vi "Parse Next XML Tag.vi"(8 "error in (no error)":errorcluster, 11 "XML in":string) -> (0 "error out":errorcluster, 1 "Tag":string, 2 "Before Tag":string, 3 "XML out":string)   [LabVIEW 2017, in "Feed.lvclass"]
uses:
  <vilib>/NI_RSS/Feed/Feed.lvclass
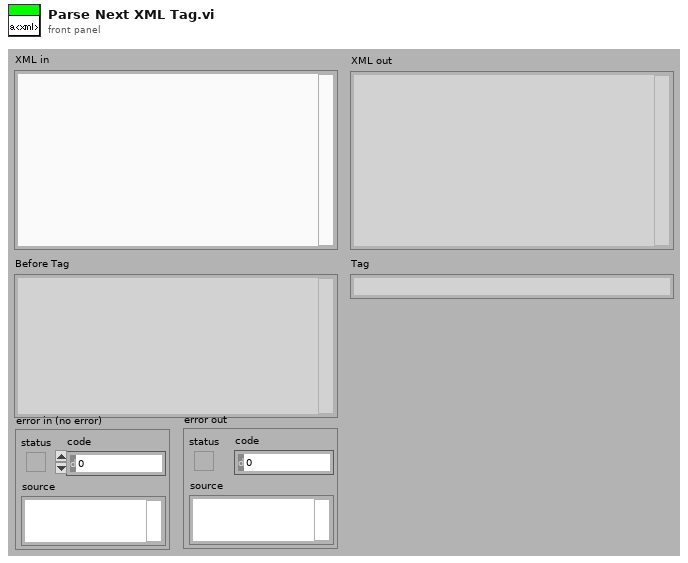
[diagram p1: front panel]
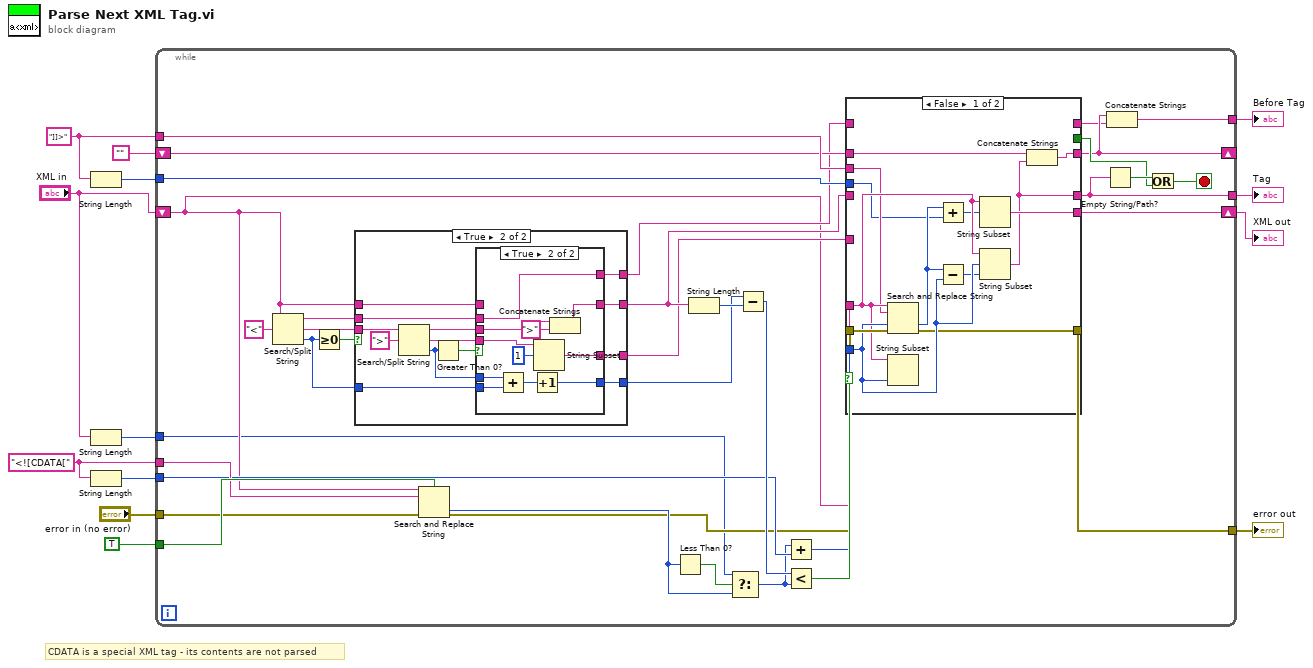
[diagram p0: block diagram]
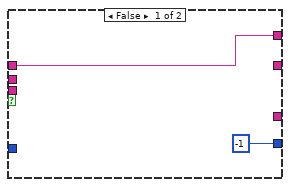
[diagram p2: hidden frame]
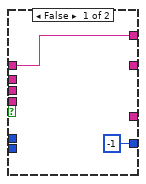
[diagram p3: hidden frame]
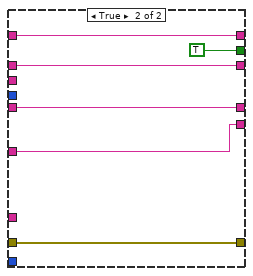
[diagram p4: hidden frame]
diagram:
  w4 = "]]>" ("regular expression")
  w6 = "<![CDATA[" ("regular expression")
  # "CDATA is a special XML tag - its contents are not parsed"
  n1 = String Length(string=w4) -> (length=w3:i32)
  n2 = String Length(string="XML in") -> (length=w1:i32)
  n3 = String Length(string=w6) -> (length=w5:i32)
  n4 = while {
    tunnel: TRUE ("ignore case? (F)") -> [w48]
    tunnel: w6 -> [w36]
    tunnel: "error in (no error)" -> [w46]
    tunnel: [w32] -> w11
    tunnel: [w41] -> w10
    tunnel: [w42] -> w8
    shift-right: [w43] -> w9
    shift-left: "XML in" -> [w15]
    shift-right: [w34] -> _
    shift-left: "" -> [w35]
    tunnel: w4 -> [w37]
    tunnel: w5 -> [w31]
    tunnel: w3 -> [w29]
    tunnel: w1 -> [w14]
    stop <- w38 stop-if-true
    n5 = Search/Split String(string=w15, search string/char (-)="<") -> (substring before match=w21:string, match + rest of string=w22:string, offset of match=w20:i32)  [unwired: 1 in]
    n6 = Greater Or Equal To 0?(x=w20) -> (x >= 0?=w23:bool)
    n7 = case shown="True" w23 {
      tunnel: w22 -> [_ w63]
      tunnel: w21 -> [_ w57]
      tunnel: w15 -> [w50 w58]
      tunnel: [_ w54] -> w18
      tunnel: [w50 w56] -> w19
      tunnel: [_ w55] -> w17
      tunnel: w20 -> [_ w52]
      tunnel: [-1 w51] -> w16
      frame False {
      }
      frame True {
        n8 = Search/Split String(string=w63, search string/char (-)=">") -> (substring before match=w59:string, match + rest of string=w60:string, offset of match=w53:i32)  [unwired: 1 in]
        n9 = Greater Than 0?(x=w53) -> (x > 0?=w61:bool)
        n10 = case shown="True" w61 {
          tunnel: w60 -> [_ w75]
          tunnel: w59 -> [_ w72]
          tunnel: w58 -> [w65 _]
          tunnel: w57 -> [_ w76]
          tunnel: [w65 w76] -> w56
          tunnel: [_ w73] -> w55
          tunnel: [_ w70] -> w54
          tunnel: w53 -> [_ w68]
          tunnel: w52 -> [_ w67]
          tunnel: [-1 w66] -> w51
          frame False {
          }
          frame True {
            n11 = Add(x=w68, y=w67) -> (x+y=w69:i32)
            n12 = Increment(x=w69) -> (x+1=w66:i32)
            n13 = String Subset(string=w75, offset (0)=1) -> (substring=w73:string)  [unwired: 1 in]
            n14 = Concatenate Strings(w72, ">" ("string")) -> (w70:string)
          }
        }
      }
    }
    n15 = Search and Replace String(case sensitive?=w48, input string=w15, search string=w36, error in=w46) -> (offset past replacement=w26:i32, error out=w25:errorcluster)  [unwired: 6 out]
    n16 = Less Than 0?(x=w26) -> (x < 0?=w27:bool)
    n17 = String Length(string=w18) -> (length=w47:i32)
    n18 = Select(t=w14, s=w27, f=w26) -> (s? t:f=w28:i32)
    n19 = Subtract(x=w16, y=w47) -> (x-y=w45:i32)
    n20 = Add(x=w28, y=w31) -> (x+y=w30:i32)
    n21 = Less?(x=w45, y=w28) -> (x < y?=w44:bool)
    n22 = case shown="False" w44 {
      tunnel: w19 -> [_ w95]
      tunnel: w18 -> [_ w94]
      tunnel: w17 -> [_ w93]
      tunnel: [_ w95] -> w33
      tunnel: [w81 w94] -> w41
      tunnel: [w82 w93] -> w43
      tunnel: w30 -> [w88 _]
      tunnel: w15 -> [w87 _]
      tunnel: w25 -> [w89 w92]
      tunnel: [w85 w92] -> w42
      tunnel: [_ TRUE] -> w39
      tunnel: w37 -> [w84 _]
      tunnel: w35 -> [w83 w90]
      tunnel: [w80 w90] -> w34
      tunnel: w29 -> [w77 _]
      frame False {
        n23 = Search and Replace String(input string=w87, search string=w84, offset=w88, error in=w89) -> (offset past replacement=w86:i32, error out=w85:errorcluster)  [unwired: 6 out]
        n24 = String Subset(string=w87, length (rest)=w88) -> ()  [unwired: 2 out]
        n25 = Add(x=w86, y=w77) -> (x+y=w78:i32)
        n26 = Subtract(x=w86, y=w88) -> (x-y=w79:i32)
        n27 = String Subset(string=w87, offset (0)=w78) -> (substring=w82:string)  [unwired: 1 out]
        n28 = String Subset(string=w87, offset (0)=w88, length (rest)=w79) -> (substring=w81:string)
        n29 = Concatenate Strings(w83, w81) -> (w80:string)
      }
      frame True {
      }
    }
    n30 = Empty String/Path?(string/path=w41) -> (empty?=w40:bool)
    n31 = Concatenate Strings(w34, w33) -> (w32:string)
    n32 = Or(x=w40, y=w39) -> (x .or. y?=w38:bool)
  }
  "XML out" <- w9
  "Before Tag" <- w11
  "Tag" <- w10
  "error out" <- w8
